vi "daqio_Get_All_Device_Channels.vi"(8 "error in (no error)":errorcluster, 11 "daq.io type in":T2={"daq.io ref"=refnum, "daq.io API Base"="http://dashboard.daq.io/api/v1", "Device Key"="", "Account ID"="", "online"=TRUE, "SSL"=TRUE}) -> (0 "error out":errorcluster, 2 "Device Channels":T1[](array[typedef]), 3 "daq.io type out":T2={"daq.io ref"=refnum, "daq.io API Base"="http://dashboard.daq.io/api/v1", "Device Key"="", "Account ID"="", "online"=TRUE, "SSL"=TRUE})   [LabVIEW 2013, in "daqio minimal.lvlib"]
doc: "This VI returns all Channel Types for a specific Device Type."
uses:
  daqio minimal.lvlib
  _typedefs/daqio-Type.ctl
  <vilib>/httpClient/ClientHandle.ctl
  _typedefs/daqio-Channels.ctl
  _typedefs/daqio-Device.ctl
  <vilib>/Easy HTTP Client/Easy HTTP.lvlib
  <vilib>/httpClient/LabVIEWHTTPClient.lvlib
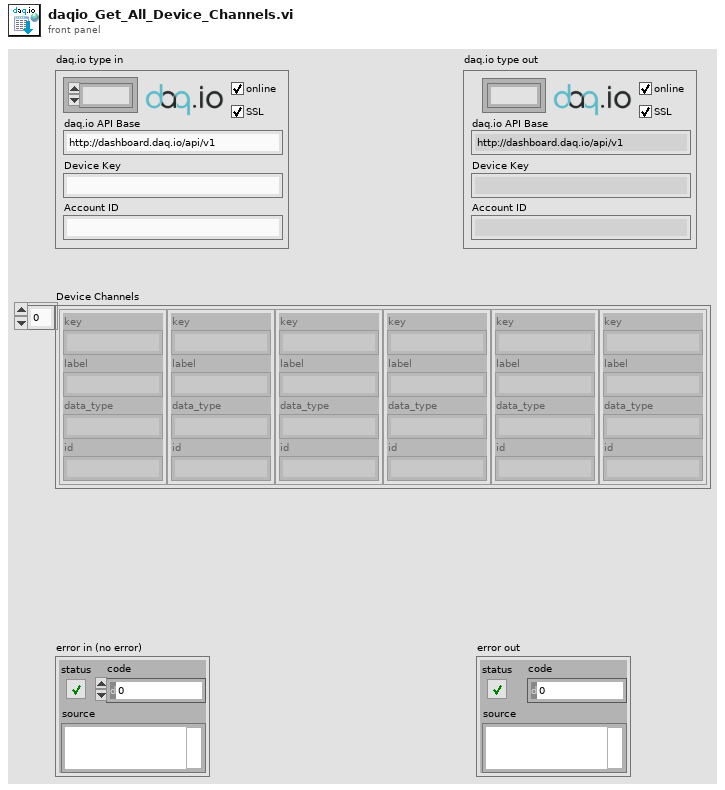
[diagram p1: front panel]
types:
  T1 = typedef "daqio minimal.lvlib/daqio-Channels.ctl" = cluster{"key":string, "label":string, "data_type":string, "id":string}
  T2 = typedef "daqio minimal.lvlib/daqio-Type.ctl" = cluster{"daq.io ref":T3, "daq.io API Base":string, "Device Key":string, "Account ID":string, "online":bool, "SSL":bool}
  T3 = typedef "LabVIEWHTTPClient.lvlib/ClientHandle.ctl" = refnum<k1>
  T4 = typedef "daqio minimal.lvlib/daqio-Device.ctl" = cluster{"id":string, "label":string, "key":string, "channels":T1[], "tags":cluster{"key":string, "value":string}[], "events":cluster{"id":string, "key":string, "label":string}[], "files":string[], "permissions":cluster{"write":string[], "read":string[]}, "dashboard":string}
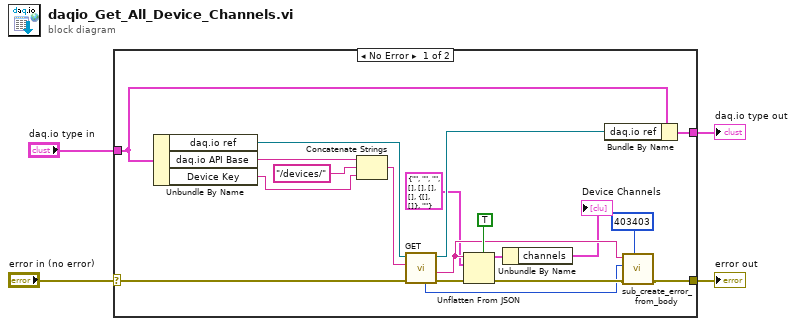
[diagram p0: block diagram]
diagram:
  n1 = case shown="No Error" "error in (no error)" {
    selector: "error in (no error)" -> [w17 w24]
    tunnel: "daq.io type in" -> [w22 w25]
    tunnel: [w21 w25] -> w3
    tunnel: [w12 w24] -> w2
    frame No Error {
      n2 = Unbundle By Name(w22) -> ("daq.io ref"=w19:T3, "daq.io API Base"=w20:string, "Device Key"=w8:string)
      n3 = Concatenate Strings(w20, "/devices/", w8) -> (w15:string)
      n4 = call <vilib>:"GET.vi"("error in (no error)"=w17, "url"=w15, "client handle"=w19) -> ("error out"=w16:errorcluster, "body"=w9:string, "client handle out"=w18:T3, "HTTP Response Code"=w10:i32)  [unwired: 4 in, 1 out]
      n5 = Unflatten From JSON(enable LabVIEW extensions? (T)=TRUE, JSON string=w9, type and defaults=T4 {"id"="", "label"="", "key"="", "channels"=[], "tags"=[], "events"=[], "files"=[], "permissions"={"write"=[], "read"=[]}, "dashboard"=""} ("Device"), error in (no error)=w16) -> (value=w6:T4, error out=w13:errorcluster)  [unwired: 3 in]
      n6 = Unbundle By Name(w6) -> ("channels"=→"Device Channels":T1[])
      n7 = Bundle By Name(cluster=w22, "daq.io ref"=w18) -> (w21:T2)
      n8 = call "sub_create_error_from_body.vi"("error code"=403403, "error in (no error)"=w13, "http code"=w10, "body"=w9) -> ("error out"=w12:errorcluster)  [unwired: 7 in]
    }
    frame Error {
    }
  }
  "error out" <- w2
  "daq.io type out" <- w3
